vi "grab trace and save to 2D arrray.vi"(8 "error in (no error)":errorcluster, 11 "VISA in":refnum<visa-resource-name>) -> (0 "error out":errorcluster, 3 "VISA out":refnum<visa-resource-name>)   [LabVIEW 2016]
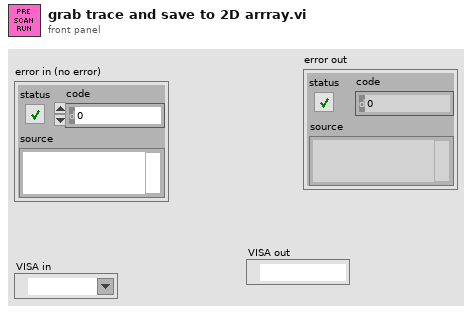
[diagram p1: front panel]
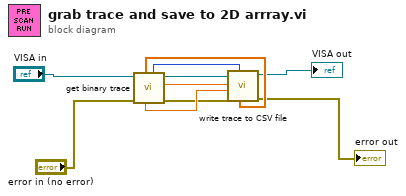
[diagram p0: block diagram]
diagram:
  n1 = call "get binary trace.vi"("error in (no error)"="error in (no error)", "VISA resource in"="VISA in") -> ("error out"=w4:errorcluster, "Start frequency (MHz)"=w10:dbl, "VISA resource out"=w6:refnum<visa-resource-name>, "Number of points"=w7:i32, "Linear frequecny increment (MHz)"=w8:dbl, "Trace Array (1D)"=w5:dbl[])  [unwired: 2 in, 1 out]
  n2 = call "write trace to CSV file.vi"("Input array"=w5, "Number of points"=w7, "error in (no error)"=w4, "Linear Increment (MHz)"=w8, "Start F (MHz)"=w10, "Visa in"=w6) -> ("error out"=→"error out":errorcluster, "VISA resource name"=→"VISA out":refnum<visa-resource-name>)  [unwired: 1 in, 3 out]
